vi "DDS RAM Programmer.vi"(6 "channel number (1)":u8=1 min=1 max=4 step=1, 8 "error in (no error)":errorcluster, 10 "RAM Word Array":u32[](array[numeric]), 11 "DDS ref in":T1={"NI USB-8451 device reference"="", "DIO port"=0, "Serial Clock Rate [kHz]"=1000}) -> (0 "error out":errorcluster, 3 "DDS ref out":T1={"NI USB-8451 device reference"="", "DIO port"=0, "Serial Clock Rate [kHz]"=1000})   [LabVIEW 2015, in "DDS.lvlib"]
doc: "This VI sends the data from an array to the RAM memory of the DDS board. The correct profile needs to be selected by the PROFILE pins before executing this VI. Also the RAM Profiles should already be programmed so the DDS board knows where to store the data."
uses:
  DDS.lvlib
  Controls/DDS Box Device Reference.ctl
  <vilib>/ni845x/ni845x.llb/ni845xControl.ctl
  Controls/AD9910 registers.ctl
panel:
  out "Read data":u8[](array[numeric])
  out "RAM Data":u8[][](array[numeric])
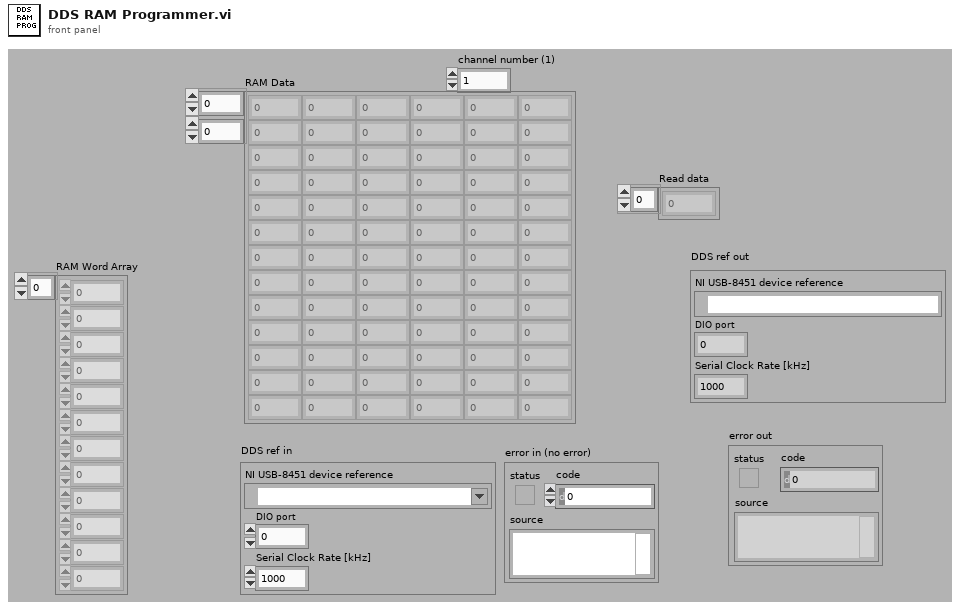
[diagram p1: front panel]
types:
  T1 = typedef "DDS.lvlib/DDS Box Device Reference.ctl" = cluster{"NI USB-8451 device reference":T2, "DIO port":u8, "Serial Clock Rate [kHz]":u16}
  T2 = typedef "ni845xControl.ctl" = refnum<k21>
  T3 = typedef "DDS.lvlib/AD9910 registers.ctl" = enum16{"CFR1", "CFR2", "CFR3", "Auxiliary DAC Control", "I/0 Update Rate", "Frequency Tuning Word", "Phase Offset Word", "Amplitude Scale Factor", "Multichip Sync", "Digital Ramp Limit", "Digital Ramp Step Size", "Digital Ramp Rate", "Single Tone Profile 0", "Single Tone Profile 1", "Single Tone Profile 2", "Single Tone Profile 3", "Single Tone Profile 4", "Single Tone Profile 5", "Single Tone Profile 6", "Single Tone Profile 7", "RAM Profile 0", "RAM Profile 1", "RAM Profile 2", "RAM Profile 3", "RAM Profile 4", "RAM Profile 5", "RAM Profile 6", "RAM Profile 7", "RAM"}
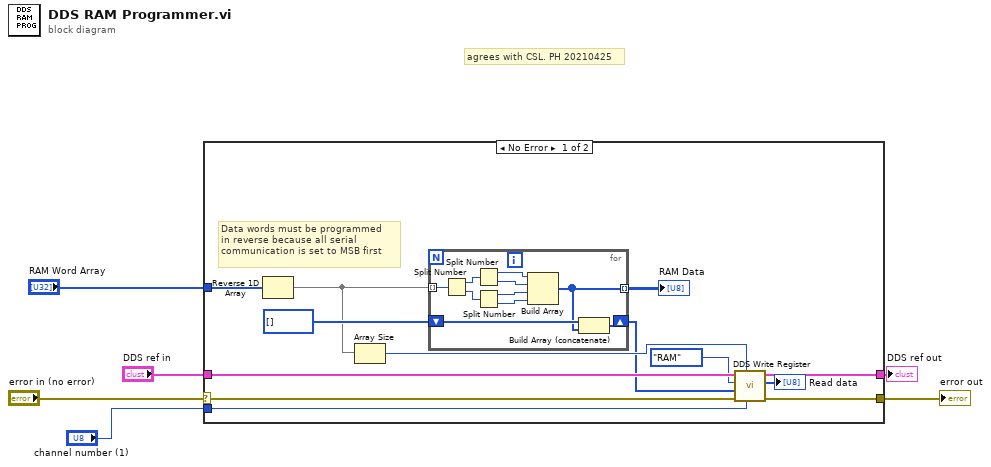
[diagram p0: block diagram]
diagram:
  # "agrees with CSL. PH 20210425"
  n1 = case shown="No Error" "error in (no error)" {
    selector: "error in (no error)" -> [w16 w30]
    tunnel: "DDS ref in" -> [w17 w31]
    tunnel: [w13 w30] -> w4
    tunnel: [w11 w31] -> w3
    tunnel: "channel number (1)" -> [w12 _]
    tunnel: "RAM Word Array" -> [w19 _]
    frame No Error {
      # "Data words must be programmed\nin reverse because all serial\ncommunication is set to MSB first"
      n2 = Reverse 1D Array(array=w19) -> (reversed array=w15:u32[])
      n3 = Array Size(array=w15) -> (size(s)=w9:i32)
      n4 = for {
        tunnel: w15 -> [w23] mode=indexing
        shift-right: [w21] -> w8
        shift-left: u8[] [] ("appended array") -> [w22]
        tunnel: [w20] -> w14 mode=indexing
        n5 = Split Number(x=w23) -> (hi(x)=w29:u16, lo(x)=w28:u16)
        n6 = Split Number(x=w29) -> (hi(x)=w24:u8, lo(x)=w25:u8)
        n7 = Split Number(x=w28) -> (hi(x)=w26:u8, lo(x)=w27:u8)
        n8 = Build Array(w24, w25, w26, w27) -> (w20:u8[])
        n9 = Build Array (concatenate)(w22, w20) -> (w21:u8[])
      }
      "RAM Data" <- w14
      n10 = call "DDS Write Register.vi"("channel number (1)"=w12, "# RAM words (0)"=w9, "error in (no error)"=w16, "Write Data"=w8, "Register"=AD9910_registers."RAM", "DDS ref in"=w17) -> ("error out"=w13:errorcluster, "Read data"=→"Read data":u8[], "DDS ref out"=w11:T1)  [unwired: 3 in]
    }
    frame Error {
    }
  }
  "error out" <- w4
  "DDS ref out" <- w3
